vi "Camera Gain_Luan2024.05.01.vi"(8 "error in (no error)":errorcluster, 10 "x":dbl, 11 "Refnum in":T1) -> (0 "error out":errorcluster, 3 "Refnum out":T1, 4 "Gain (Out) [dB]":dbl)   [LabVIEW 2023]
uses:
  <vilib>/userDefined/High Color/IMAQdx.ctl
  <resource>/objmgr/imaqdx.rc
  <vilib>/vision/driver/NI_Vision_Acquisition_Software.lvlib
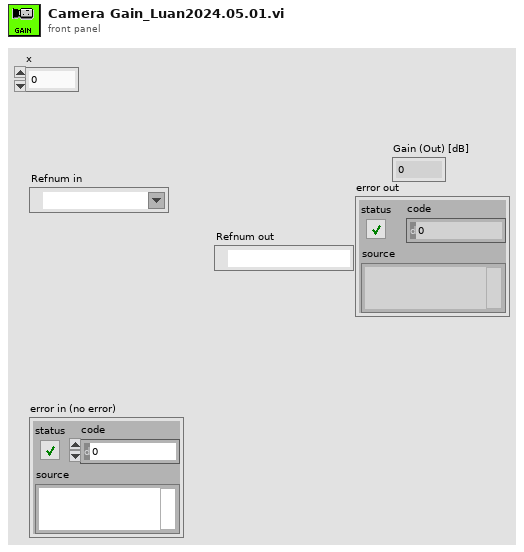
[diagram p1: front panel]
types:
  T1 = typedef "IMAQdx.ctl" = refnum<k21>
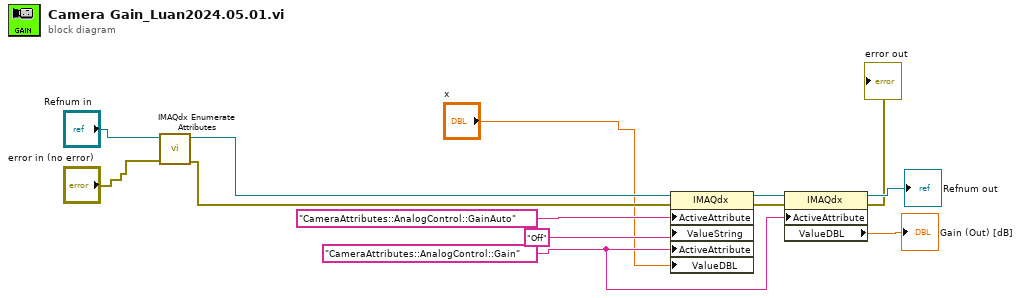
[diagram p0: block diagram]
diagram:
  w6 = "CameraAttributes::AnalogControl::Gain" ("ActiveAttribute")
  n1 = call <vilib>:"IMAQdx Enumerate Attributes.vi"("error in"="error in (no error)", "Session In"="Refnum in") -> ("error out"=w3:errorcluster, "Session Out"=w4:T1)  [unwired: 7 in, 1 out]
  n2 = property class="IMAQdx"(reference=w4, error in=w3, "ActiveAttribute"="CameraAttributes::AnalogControl::GainAuto", "ValueString"="Off", "ActiveAttribute"=w6, "ValueDBL"="x") -> (reference out=w11:T1, error out=w10:errorcluster)
  n3 = property class="IMAQdx"(reference=w11, error in=w10, "ActiveAttribute"=w6) -> (reference out=→"Refnum out":T1, error out=→"error out":errorcluster, "ValueDBL"=→"Gain (Out) [dB]":dbl)
